vi "CreateDataFlowMaps.vi"(8 "error in (no error)":errorcluster, 10 "settling time met":bool, 11 "MCSA Acquisition Config":T1 {"FixedSizeX31"."InputConfig" items=["AC Coupled", "DC Coupled", "IEPE AC Coupled"]}) -> (0 "error out":errorcluster, 1 "maps":T8[](array[typedef]), 3 "MCSA Acquisition Config out":T1 {"FixedSizeX31"."InputConfig" items=["AC Coupled", "DC Coupled", "IEPE AC Coupled"]})   [LabVIEW 2017, in "McsaFpgaAcquisition.lvlib"]
uses:
  <vilib>/addons/InsightCM/Devices/Shared/Mcsa/McsaFpgaAcquisition/McsaFpgaAcquisition.lvlib
  <vilib>/addons/InsightCM/Devices/Shared/Mcsa/McsaFpgaAcquisition/controls/Configuration.ctl
  <vilib>/addons/InsightCM/Devices/Shared/Cms/CmsAcquisition/controls/FixedSizeArrays.ctl
  <vilib>/LabVIEW Targets/FPGA/cRIO/shared/nicrio_ModuleControls/nicrio_cRIO-9232_ConfigModeRing.ctl
  <vilib>/addons/InsightCM/Devices/Shared/Cms/cRIOWfmAcq/subVIs/RIO Wfm Cust Ctrls/rwfm_SamplingInfo.ctl
  <vilib>/addons/InsightCM/Devices/Shared/Mcsa/McsaFpgaAcquisition/controls/Group.ctl
  <vilib>/addons/InsightCM/Devices/Shared/Mcsa/McsaFpgaAcquisition/controls/ChannelMcsa.ctl
  <vilib>/addons/InsightCM/Devices/Shared/Mcsa/McsaFpgaAcquisition/controls/RangeParams.ctl
  <vilib>/addons/PointValueMap/controls/PointMap.ctl
  <vilib>/addons/PointValueMap/subVIs/Point_Write_double.vi
  <vilib>/addons/PointValueMap/subVIs/Point_Write_i32.vi
  <vilib>/addons/PointValueMap/PointValueMap.lvlib
  <vilib>/addons/InsightCM/Devices/Shared/Cms/cRIOWfmAcq/cRIOWfmLib.lvlib
  <vilib>/addons/InsightCM/Devices/Shared/Cms/CmsAcquisition/CmsAcquisition.lvlib
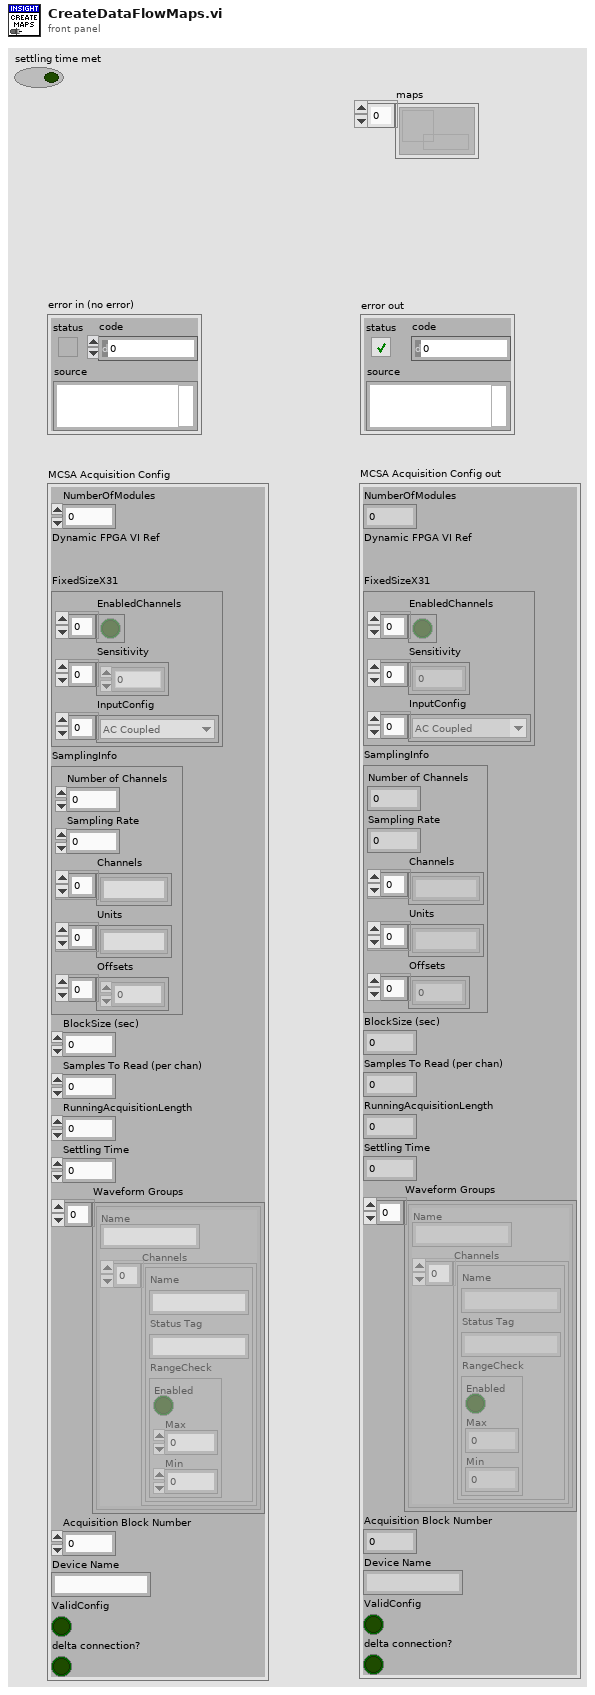
[diagram p1: front panel]
types:
  T1 = typedef "McsaFpgaAcquisition.lvlib/Configuration.ctl" = cluster{"NumberOfModules":i16, "Dynamic FPGA VI Ref":refnum<k20>, "FixedSizeX31":T2, "SamplingInfo":T4, "BlockSize (sec)":dbl, "Samples To Read (per chan)":i32, "RunningAcquisitionLength":dbl, "Settling Time":dbl, "Waveform Groups":T5[], "Acquisition Block Number":i32, "Device Name":string, "ValidConfig":bool, "delta connection?":bool}
  T2 = typedef "CmsAcquisition.lvlib/FixedSizeArrays.ctl" = cluster{"EnabledChannels":bool[], "Sensitivity":dbl[], "InputConfig":T3[]}
  T3 = typedef "nicrio_cRIO-9232_ConfigModeRing.ctl" = u8
  T4 = typedef "cRIOWfmLib.lvlib/rwfm_SamplingInfo.ctl" = cluster{"Number of Channels":i32, "Sampling Rate":dbl, "Channels":string[], "Units":string[], "Offsets":sgl[]}
  T5 = typedef "McsaFpgaAcquisition.lvlib/Group.ctl" = cluster{"Name":string, "Channels":T6[]}
  T6 = typedef "McsaFpgaAcquisition.lvlib/ChannelMcsa.ctl" = cluster{"Name":string, "Status Tag":string, "RangeCheck":T7}
  T7 = typedef "McsaFpgaAcquisition.lvlib/RangeParams.ctl" = cluster{"Enabled":bool, "Max":dbl, "Min":dbl}
  T8 = typedef "PointValueMap.lvlib/PointMap.ctl" = refnum<data-value>
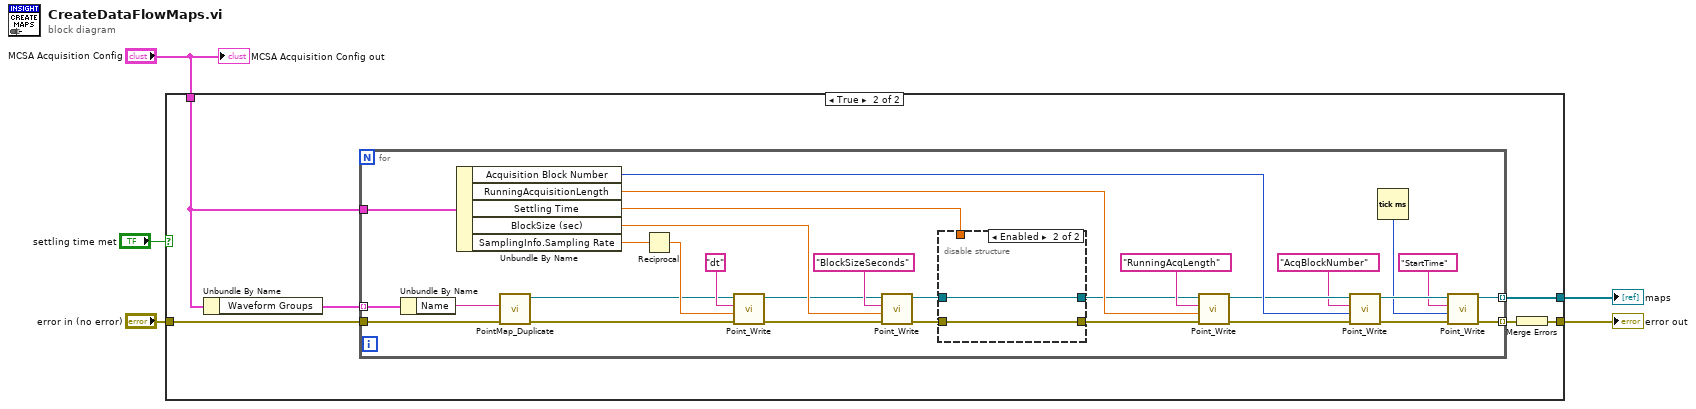
[diagram p0: block diagram]
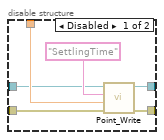
[diagram p3: hidden frame]
diagram:
  n1 = case shown="True" "settling time met" {
    tunnel: [w6 w12] -> w5
    tunnel: "error in (no error)" -> [w6 w10]
    tunnel: "MCSA Acquisition Config" -> [_ w9]
    tunnel: [_ w7] -> w2
    frame False {
    }
    frame True {
      n2 = Unbundle By Name(w9) -> ("Waveform Groups"=w11:T5[])
      n3 = for {
        tunnel: w11 -> [w42] mode=indexing
        tunnel: w10 -> [w40]
        tunnel: w9 -> [w21]
        tunnel: [w13] -> w8 mode=indexing
        tunnel: [w14] -> w7 mode=indexing
        n4 = Unbundle By Name(w42) -> ("Name"=w41:string)
        n5 = Unbundle By Name(w21) -> ("Acquisition Block Number"=w35:i32, "RunningAcquisitionLength"=w36:dbl, "Settling Time"=w38:dbl, "BlockSize (sec)"=w39:dbl, "SamplingInfo.Sampling Rate"=w37:dbl)
        n6 = call <vilib>:"PointMap_Duplicate.vi"("error in (no error)"=w40, "Source Map Name"=w41) -> ("error out"=w19:errorcluster, "Map Out"=w20:T8)  [unwired: 8 in]
        n7 = Reciprocal(x=w37) -> (1/x=w25:dbl)
        n8 = call-poly <vilib>:"Point_Write.vi"("Error In"=w19, "Value"=w25, "Tag"="dt", "Map"=w20) -> ("Error Out"=w27:errorcluster, "Map Out"=w26:T8)  [unwired: 6 in]
        n9 = call-poly <vilib>:"Point_Write.vi"("Error In"=w27, "Value"=w39, "Tag"="BlockSizeSeconds", "Map"=w26) -> ("Error Out"=w29:errorcluster, "Map Out"=w32:T8)  [unwired: 6 in]
        n10 = disable-structure shown="Enabled" {
          disable-tunnel: w38 -> [w48 _]
          disable-tunnel: w32 -> [w46 w50]
          disable-tunnel: [w45 w50] -> w31
          disable-tunnel: [w44 w49] -> w30
          disable-tunnel: w29 -> [w43 w49]
          frame Disabled {
            n11 = call-poly <vilib>:"Point_Write.vi"("Error In"=w43, "Value"=w48, "Tag"="SettlingTime", "Map"=w46) -> ("Error Out"=w44:errorcluster, "Map Out"=w45:T8)  [unwired: 6 in]
          }
          frame Enabled {
          }
        }
        n12 = call-poly <vilib>:"Point_Write.vi"("Error In"=w30, "Value"=w36, "Tag"="RunningAcqLength", "Map"=w31) -> ("Error Out"=w23:errorcluster, "Map Out"=w24:T8)  [unwired: 6 in]
        n13 = call-poly <vilib>:"Point_Write.vi"("Error In"=w23, "Value"=w35, "Tag"="AcqBlockNumber", "Map"=w24) -> ("Error Out"=w18:errorcluster, "Map Out"=w17:T8)  [unwired: 6 in]
        n14 = Tick Count (ms)() -> (millisecond timer value=w15:u32)
        n15 = call-poly <vilib>:"Point_Write.vi"("Error In"=w18, "Value"=w15, "Tag"="StartTime", "Map"=w17) -> ("Error Out"=w13:errorcluster, "Map Out"=w14:T8)  [unwired: 6 in]
      }
      n16 = Merge Errors(w8) -> (w12:errorcluster)
    }
  }
  "error out" <- w5
  "maps" <- w2
  "MCSA Acquisition Config out" <- "MCSA Acquisition Config"
